vi "Replace Default Text Formatting.vi"(3 "New Default Message Formatting":T1={"Font"="Consolas", "Text Color"=enum."Blue", "Text Background Color"=enum."White", "Text Style"=enum."Regular", "Font Size (Points)"=10.0, "Text Alignment"=0} {"Text Alignment" items=["Left", "Right", "Center"]}, 4 "Message Formatting in":T1={"Font"="Default", "Text Color"=enum."Unchanged", "Text Background Color"=enum."Unchanged", "Text Style"=enum."Regular", "Font Size (Points)"=-1.0, "Text Alignment"=0} {"Text Alignment" items=["Left", "Right", "Center"]}) -> (2 "Message Formatting out":T1 {"Text Alignment" items=["Left", "Right", "Center"]})   [LabVIEW 2021, in "Rich Text Box.lvlib"]
doc: "If <B>Message Formatting in</B> is the default text formatting (created using \"Use Default\" in Case Structures), replaces it by a user provided <B>New Default Message Formatting</B>."
uses:
  Rich Text Box/Text Formatting.ctl
  Rich Text Box/Text Colors.ctl
  Rich Text Box/Rich Text Box.lvlib
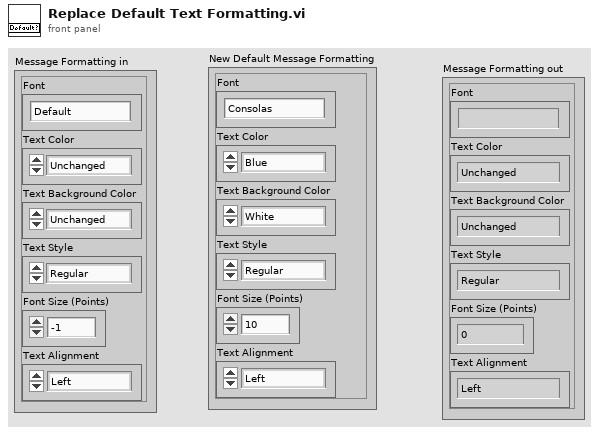
[diagram p1: front panel]
types:
  T1 = typedef "Rich Text Box.lvlib/Text Formatting.ctl" = cluster{"Font":string, "Text Color":T2, "Text Background Color":T2, "Text Style":enum16{"Regular", "Bold", "Italic", "Underline", "Strikeout"}, "Font Size (Points)":dbl, "Text Alignment":i32}
  T2 = typedef "Rich Text Box.lvlib/Text Colors.ctl" = enum16{"Unchanged", "Black", "Blue", "Brown", "Gray", "Green", "Orange", "Pink", "Red", "White"}
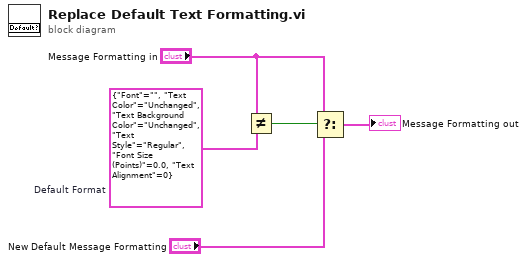
[diagram p0: block diagram]
diagram:
  w5 = T1 {"Font"="", "Text Color"=enum."Unchanged", "Text Background Color"=enum."Unchanged", "Text Style"=enum."Regular", "Font Size (Points)"=0.0, "Text Alignment"=0}  # Default Format
  n1 = Not Equal?(x="Message Formatting in", y=w5) -> (x != y?=w4:bool)
  n2 = Select(t="Message Formatting in", s=w4, f="New Default Message Formatting") -> (s? t:f=→"Message Formatting out":T1)
